vi "Set VMode.vi"(8 "error in (no error)":errorcluster, 10 "VMode (5V)":T1, 11 "Queue in":T2) -> (0 "error out":errorcluster, 3 "Queue out":T2)   [LabVIEW 2019, in "Controller.lvlib"]
uses:
  Controller.lvlib
  Controller Message Queue.ctl
  Controller Message.ctl
  MDS Command.ctl
  VMode.ctl
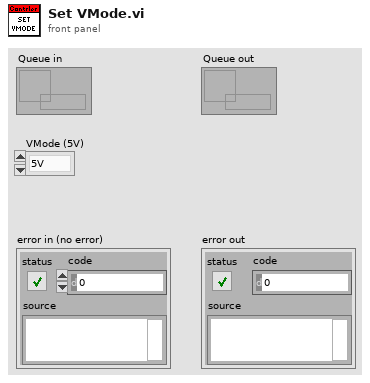
[diagram p1: front panel]
types:
  T1 = typedef "Controller.lvlib/VMode.ctl" = enum8{"5V", "10V"}
  T2 = typedef "Controller.lvlib/Controller Message Queue.ctl" = refnum<queue>
  T3 = typedef "Controller.lvlib/Controller Message.ctl" = cluster{"MDS Command":T4, "Channel":u8, "Value":variant}
  T4 = typedef "Controller.lvlib/MDS Command.ctl" = enum16{"Idle", "Open", "Set VMode", "Set IMode", "Get Frequency", "Set Frequency", "Get Power", "Set Power (dBm)", "Set Power (%)", "Get Switch", "Switch Channel", "Store", "Wait for Prompt", "Wait for State", "Reset", "Error", "Close", "Stop"}
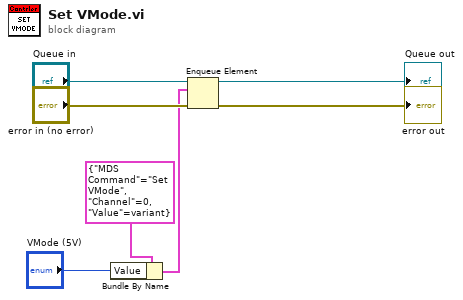
[diagram p0: block diagram]
diagram:
  n1 = Bundle By Name(cluster=T3 {"MDS Command"=enum."Set VMode", "Channel"=0, "Value"=variant} ("Controller Message"), "Value"="VMode (5V)") -> (w1:T3)
  n2 = Enqueue Element(queue="Queue in", element=w1, error in (no error)="error in (no error)") -> (queue out=→"Queue out":T2, error out=→"error out":errorcluster)  [unwired: 1 in, 1 out]
